vi "Pulse Train IsEqual.vi"(8 "related precise":dbl=1e-10, 10 "x2":dbl, 11 "x1":dbl format="%_5g") -> (3 "x1 = x2?":bool)   [LabVIEW 2017, in "NI_AALBase.lvlib"]
uses:
  NI_AALBase.lvlib
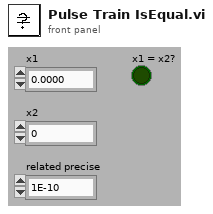
[diagram p1: front panel]
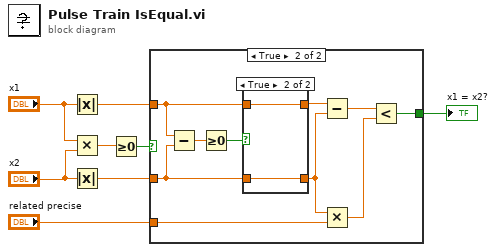
[diagram p0: block diagram]
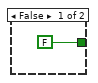
[diagram p2: hidden frame]
diagram:
  n1 = Absolute Value(x="x1") -> (abs(x)=w2:dbl)
  n2 = Multiply(x="x1", y="x2") -> (x*y=w4:dbl)
  n3 = Absolute Value(x="x2") -> (abs(x)=w1:dbl)
  n4 = Greater Or Equal To 0?(x=w4) -> (x >= 0?=w8:bool)
  n5 = case shown="True" w8 {
    tunnel: [FALSE w14] -> w7
    tunnel: "related precise" -> [_ w12]
    tunnel: w2 -> [_ w17]
    tunnel: w1 -> [_ w16]
    frame False {
    }
    frame True {
      n6 = Subtract(x=w17, y=w16) -> (x-y=w19:dbl)
      n7 = Greater Or Equal To 0?(x=w19) -> (x >= 0?=w18:bool)
      n8 = case shown="True" w18 {
        tunnel: w17 -> [w21 w23]
        tunnel: w16 -> [w20 w22]
        tunnel: [w20 w23] -> w15
        tunnel: [w21 w22] -> w13
        frame False {
        }
        frame True {
        }
      }
      n9 = Subtract(x=w15, y=w13) -> (x-y=w11:dbl)
      n10 = Multiply(x=w13, y=w12) -> (x*y=w10:dbl)
      n11 = Less?(x=w11, y=w10) -> (x < y?=w14:bool)
    }
  }
  "x1 = x2?" <- w7
